vi "ArrowHead_Create.vi"(1 "arrowHead":T1, 5 "error in (no error)":errorcluster) -> (14 "reference out":refnum<class "ArrowHead.lvclass">, 19 "error out":errorcluster)   [LabVIEW 2014, in "ArrowHead.lvclass"]
doc: "Creates and initializes a new ArrowHead object.\n\nThis object should be destroyed using a ArrowHead destructor VI.\n\n[GOOP 2.1]"
uses:
  <resource>/Framework/Providers/Open_GDS/UML/ArrowHead_class/ArrowHead.lvclass
  <resource>/Framework/Providers/Open_GDS/UML/ArrowHead_class/ArrowHeadType.ctl
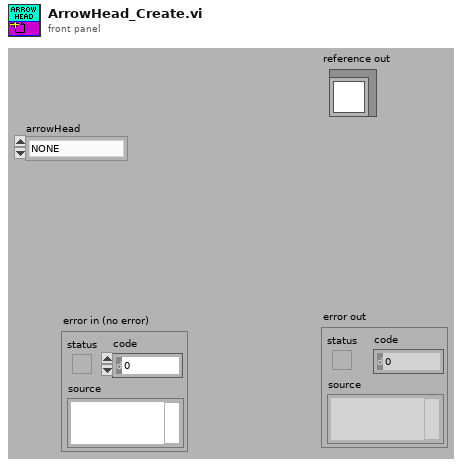
[diagram p1: front panel]
types:
  T1 = typedef "ArrowHead.lvclass/ArrowHeadType.ctl" = enum16{"NONE", "TRIANGLE", "BLACK_TRIANGLE", "V", "HALF_V", "DIAMOND", "BLACK_DIAMOND"}
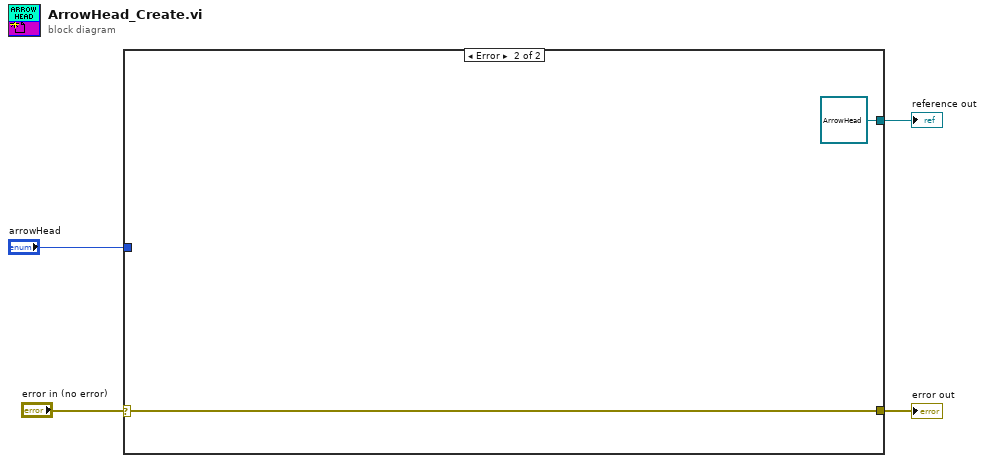
[diagram p0: block diagram]
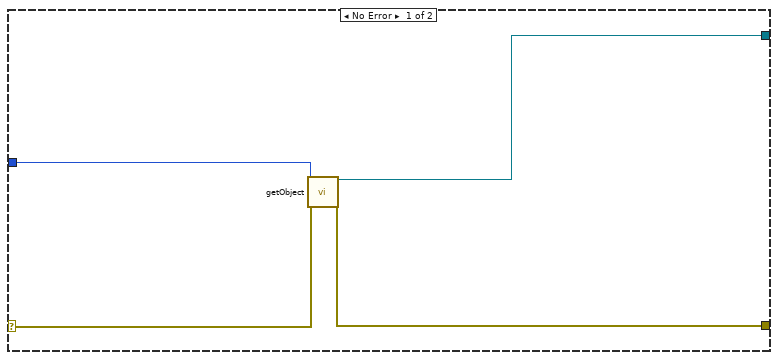
[diagram p2: hidden frame]
diagram:
  n1 = case shown="Error" "error in (no error)" {
    selector: "error in (no error)" -> [w5 w10]
    tunnel: [w7 refnum<class "ArrowHead.lvclass"> refnum ("reference out")] -> w4
    tunnel: [w6 w10] -> w3
    tunnel: "arrowHead" -> [w8 _]
    frame No Error {
      n2 = call <resource>:"getObject.vi"("arrowHead"=w8, "error in (no error)"=w5) -> ("reference out"=w7:refnum<class "ArrowHead.lvclass">, "error out"=w6:errorcluster)  [unwired: 16 in]
    }
    frame Error {
    }
  }
  "error out" <- w3
  "reference out" <- w4
